vi "CRYSet Add curve Front Panel.vi"(11 "Vi Ref":refnum<vi>) -> ()   [LabVIEW 2013]
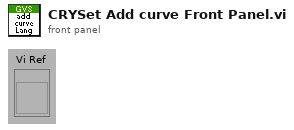
[diagram p1: front panel]
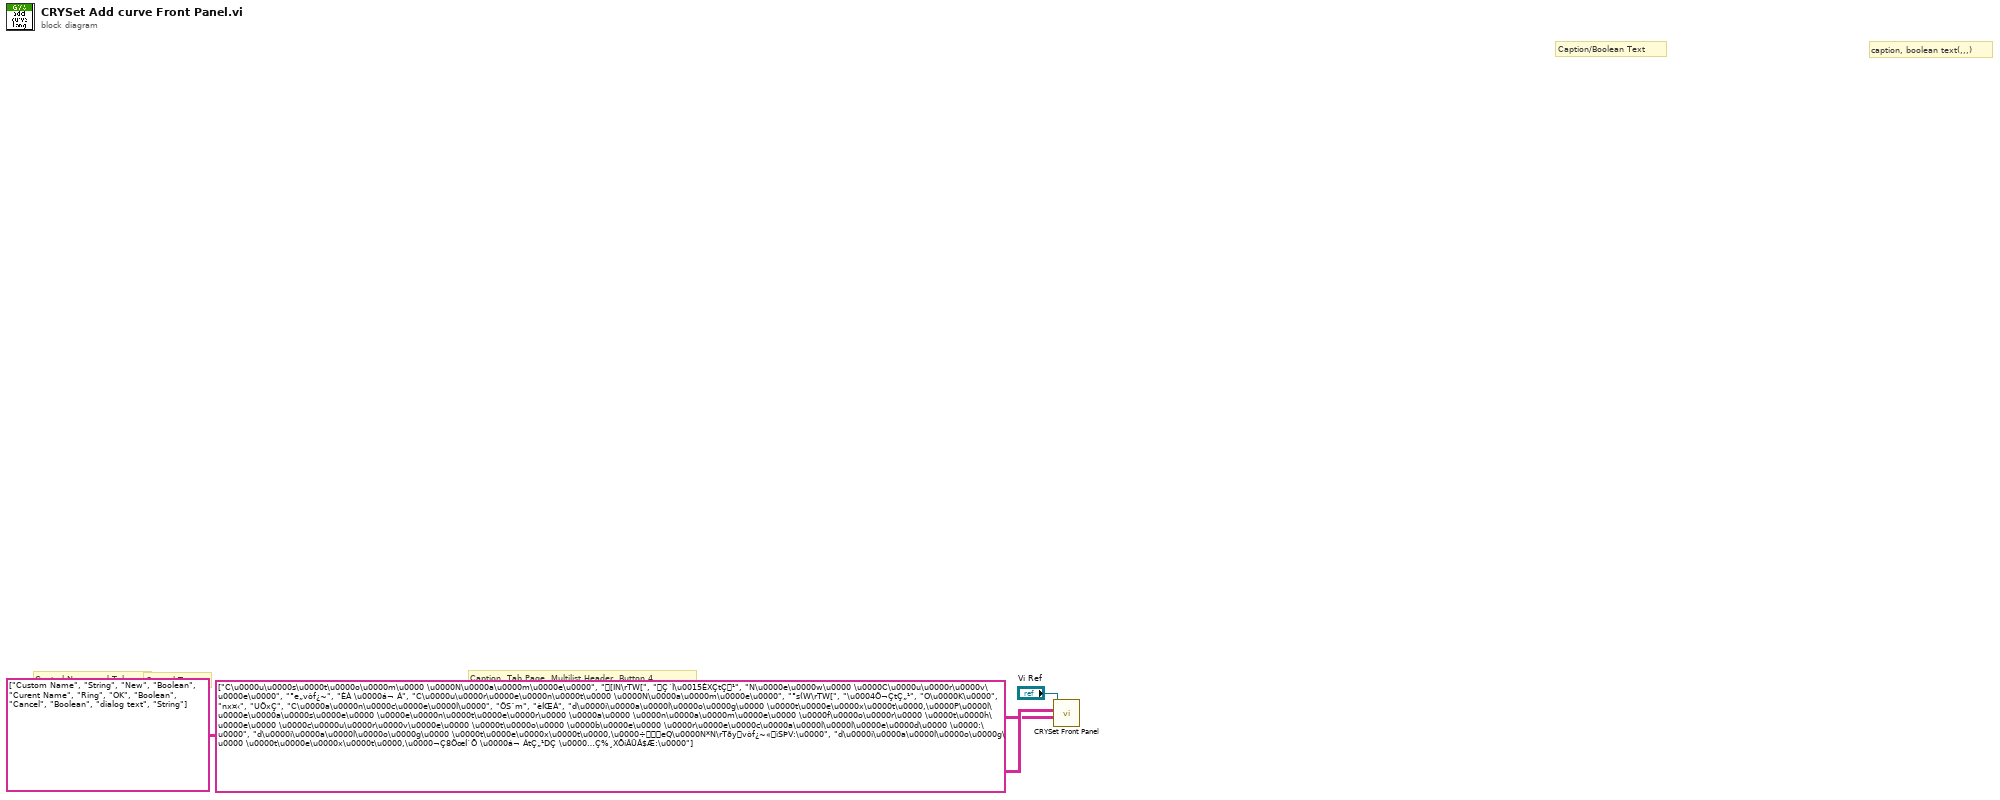
[diagram p0: block diagram]
diagram:
  # "Caption, Tab Page, Multilist Header, Button 4"
  # "Control Type"
  # "Control Name and Tab"
  # "caption, boolean text(,,,)"
  # "Caption/Boolean Text"
  n1 = call "CRYSet Front Panel.vi"("Caption(Boolean Text)"=string[][] [["C\u0000u\u0000s\u0000t\u0000o\u0000m\u0000 \u0000N\u0000a\u0000m\u0000e\u0000", "ꁚ[IN\rTW[", "Ç´Ì\u0015ÈXÇtÇ¹"], ["N\u0000e\u0000w\u0000 \u0000C\u0000u\u0000r\u0000v\u0000e\u0000", "°e„vòf¿~", "ÈÀ \u0000á¬ Á"], ["C\u0000u\u0000r\u0000e\u0000n\u0000t\u0000 \u0000N\u0000a\u0000m\u0000e\u0000", "°s(W\rTW[", "\u0004Ö¬ÇtÇ„¹"], ["O\u0000K\u0000", "nx¤‹", "UÖxÇ"], ["C\u0000a\u0000n\u0000c\u0000e\u0000l\u0000", "ÖSˆm", "èÍŒÁ"], ["d\u0000i\u0000a\u0000l\u0000o\u0000g\u0000 \u0000t\u0000e\u0000x\u0000t\u0000,\u0000P\u0000l\u0000e\u0000a\u0000s\u0000e\u0000 \u0000e\u0000n\u0000t\u0000e\u0000r\u0000 \u0000a\u0000 \u0000n\u0000a\u0000m\u0000e\u0000 \u0000f\u0000o\u0000r\u0000 \u0000t\u0000h\u0000e\u0000 \u0000c\u0000u\u0000r\u0000v\u0000e\u0000 \u0000t\u0000o\u0000 \u0000b\u0000e\u0000 \u0000r\u0000e\u0000c\u0000a\u0000l\u0000l\u0000e\u0000d\u0000 \u0000:\u0000", "d\u0000i\u0000a\u0000l\u0000o\u0000g\u0000 \u0000t\u0000e\u0000x\u0000t\u0000,\u0000÷eQ\u0000N*N\rTðyvòf¿~«ìSÞV:\u0000", "d\u0000i\u0000a\u0000l\u0000o\u0000g\u0000 \u0000t\u0000e\u0000x\u0000t\u0000,\u0000¬Ç8ÖœÍ`Õ \u0000á¬ ÁtÇ„¹DÇ \u0000…Ç%¸XÕíÂÜÂ$Æ:\u0000"]], "Control ID and Type(Label Name, Type)"=string[][] [["Custom Name", "String"], ["New", "Boolean"], ["Curent Name", "Ring"], ["OK", "Boolean"], ["Cancel", "Boolean"], ["dialog text", "String"]], "Vi Ref"="Vi Ref") -> ()  [unwired: 9 in]
